vi "UnitTest - Backup Functionality.vi"(8 "error in (no error)":errorcluster) -> (0 "error out":errorcluster)   [LabVIEW 2014]
uses:
  TableLogger_Actor/TableLoggerConfig.ctl
  TableLogger_Actor/TableLoggerTypes.ctl
  TableLogger_Actor/TableLoggerBackupConfig.ctl
  <vilib>/addons/_JKI Toolkits/Caraya/classes/Test Suite/Test Suite.lvclass
  TableLogger_Actor/TableLogger_Actor.lvlib
panel:
  # "Connector Pane"
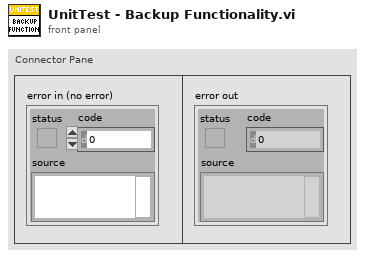
[diagram p1: front panel]
types:
  T1 = typedef "TableLogger_Actor.lvlib/TableLoggerConfig.ctl" = cluster{"TableLogger":T2, "DB File Path":path, "DB Backup Config":T3}
  T2 = typedef "TableLogger_Actor.lvlib/TableLoggerTypes.ctl" = enum16{"CSV Logger", "SQLite Logger"}
  T3 = typedef "TableLogger_Actor.lvlib/TableLoggerBackupConfig.ctl" = cluster{"Directory":path, "UTC Time Format":bool, "On Launch":bool, "Interval (Hours)":dbl, "Size Multiples (Bytes)":i32}
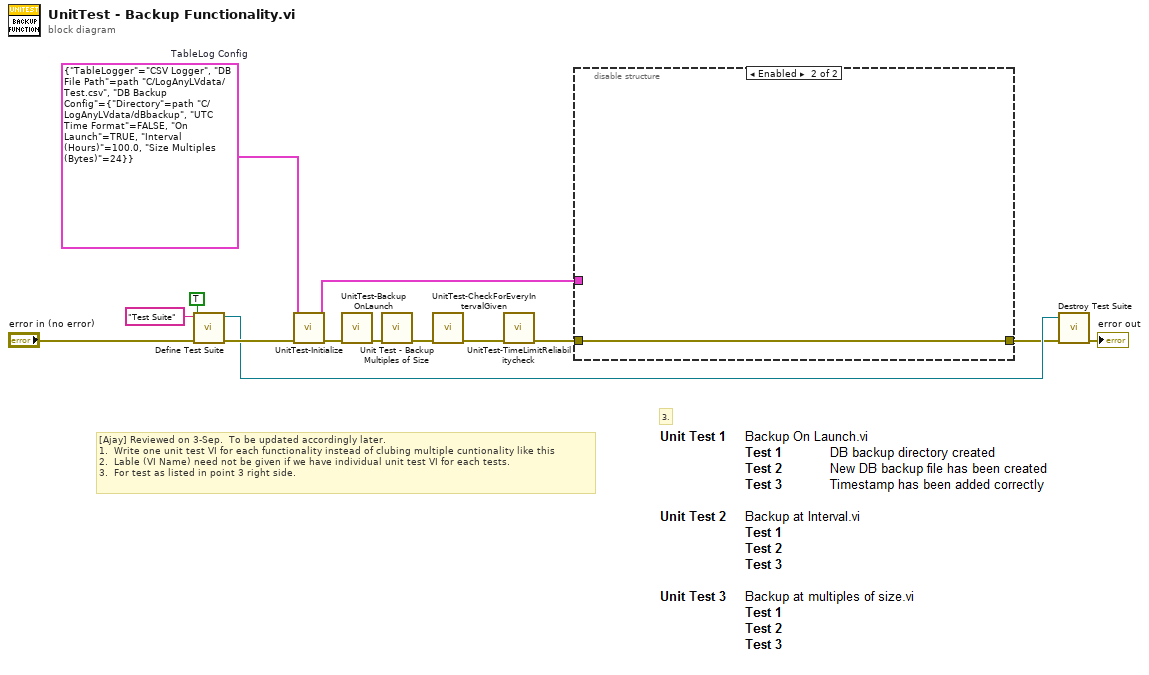
[diagram p0: block diagram]
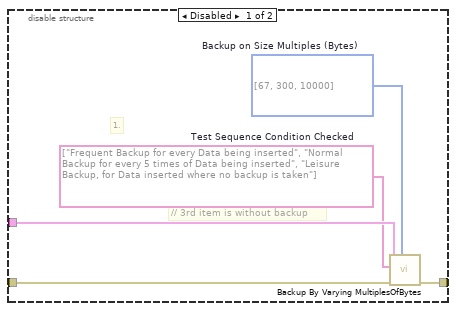
[diagram p2: hidden frame]
diagram:
  w8 = T1 {"TableLogger"=enum."CSV Logger", "DB File Path"=path "C:/LogAnyLVdata/Test.csv", "DB Backup Config"={"Directory"=path "C:/LogAnyLVdata/dBbackup", "UTC Time Format"=FALSE, "On Launch"=TRUE, "Interval (Hours)"=100.0, "Size Multiples (Bytes)"=24}}  # TableLog Config
  # "3."
  # "[Ajay] Reviewed on 3-Sep.  To be updated accordingly later.\n1.  Write one unit test VI for each functionality instead of clubing multiple cuntionality like this\n2.  Lable (VI Name) need not be given if we have individual unit test VI for each tests.\n3.  For test as listed in point 3 right side."
  n1 = call <vilib>:"Define Test Suite.vi"("error in (no error)"="error in (no error)", "Interactive"=TRUE, "Label (VI Title)"="Test Suite") -> ("error out"=w14:errorcluster, "Test Suite"=w11:refnum<class "Test Suite.lvclass">)  [unwired: 7 in]
  n2 = call "UnitTest-Initialize.vi"("error in"=w14, "Config IN"=w8) -> ("error out"=w5:errorcluster, "Config OUT"=w7:T1)  [unwired: 7 in, 1 out]
  n3 = call "UnitTest-BackupOnLaunch.vi"("error in (no error)"=w5) -> ("error out"=w4:errorcluster)  [unwired: 10 in]
  n4 = call "Unit Test - Backup Multiples of Size.vi"("error in (no error)"=w4) -> ("error out"=w3:errorcluster)  [unwired: 10 in]
  n5 = call "UnitTest-CheckForEveryIntervalGiven.vi"("error in (no error)"=w3) -> ("error out"=w2:errorcluster)  [unwired: 10 in]
  n6 = call "UnitTest-TimeLimitReliabilitycheck.vi"("error in (no error)"=w2) -> ("error out"=w1:errorcluster)  [unwired: 10 in]
  n7 = disable-structure shown="Enabled" {
    disable-tunnel: w7 -> [w19 _]
    disable-tunnel: [w18 w20] -> w6
    disable-tunnel: w1 -> [w15 w20]
    frame Disabled {
      w16 = string[] ["Frequent Backup for every Data being inserted", "Normal Backup for every 5 times of Data being inserted", "Leisure Backup, for Data inserted where no backup is taken"]  # Test Sequence Condition Checked
      w17 = i32[] [67, 300, 10000]  # Backup on Size Multiples (Bytes)
      # "1."
      # "// 3rd item is without backup"
      n8 = call "Backup By Varying MultiplesOfBytes.vi"("Backup on Size Multiples (Bytes)"=w17, "error in"=w15, "Test Sequence Condition Checked"=w16, "TableLogger Config"=w19) -> ("error out"=w18:errorcluster)  [unwired: 7 in]
    }
    frame Enabled {
    }
  }
  n9 = call-dynamic "Destroy Test Suite.vi"("error in (no error)"=w6, "Test Suite in"=w11) -> ("error out"=→"error out":errorcluster)  [unwired: 9 in]
